vi "Calculate Waveform Duration.vi"(1 "Sample Rate":dbl format="%#_6p", 5 "Burst Start Locations":i32[](array[numeric]), 9 "Burst Stop Locations":i32[](array[numeric])) -> (8 "Burst Length (s)":dbl format="%#_6p")   [LabVIEW 2019, in "SG.lvlib"]
doc: "Calculates the waveform duration between the first and final burst."
uses:
  SG.lvlib
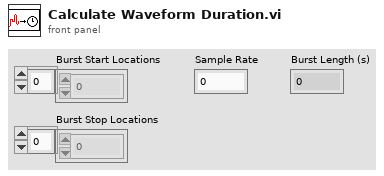
[diagram p1: front panel]
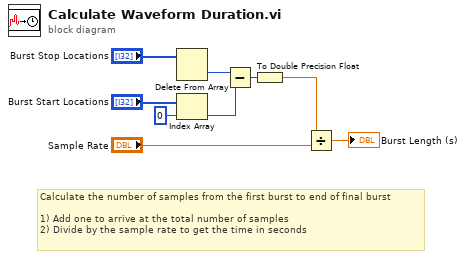
[diagram p0: block diagram]
diagram:
  # "Calculate the number of samples from the first burst to end of final burst\n\n1) Add one to arrive at the total number of samples\n2) Divide by the sample rate to get the time in seconds"
  n1 = Delete From Array(array="Burst Stop Locations") -> (deleted portion=w3:i32)  [unwired: 2 in, 1 out]
  n2 = Index Array(array="Burst Start Locations", index=0) -> (element=w2:i32)
  n3 = Subtract(x=w3, y=w2) -> (x-y=w9:i32)
  n4 = To Double Precision Float(number=w9) -> (double precision float=w1:dbl)
  n5 = Divide(x=w1, y="Sample Rate") -> (x/y=→"Burst Length (s)":dbl)
